vi "Get Tuner Gains.vi"(8 "error in (no error)":errorcluster, 11 "DeviceRefnum":u64) -> (0 "error out":errorcluster, 2 "Supported Gains":dbl[](array[numeric]), 3 "DeviceRefnum Out":u64)   [LabVIEW 2014]
doc: "Get a list of gains supported by the tuner."
panel:
  in  "Gains Buffer":i32[](array[numeric])
  out "function return":i32
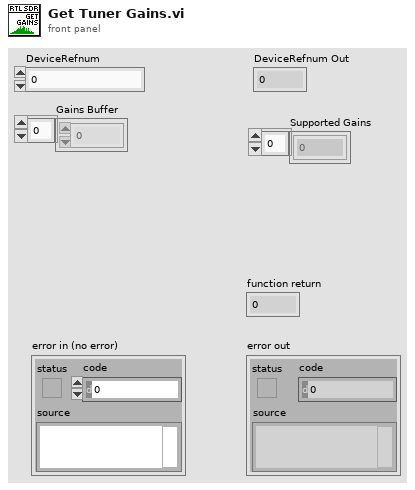
[diagram p1: front panel]
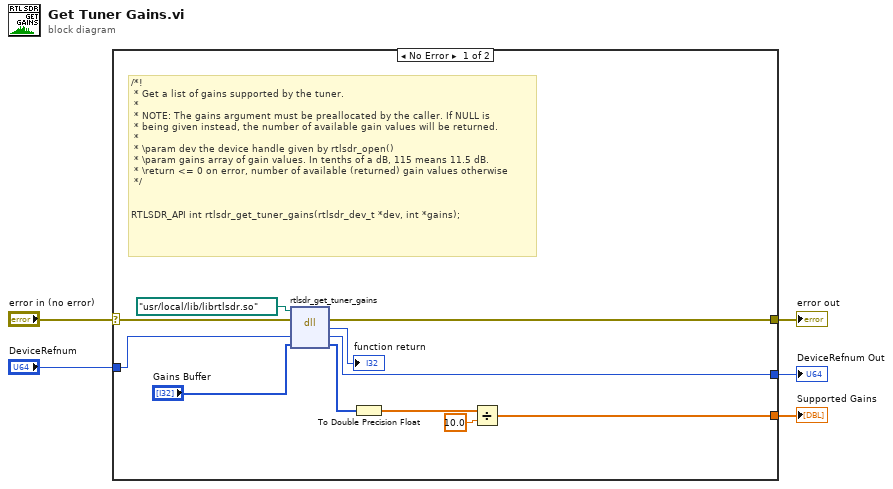
[diagram p0: block diagram]
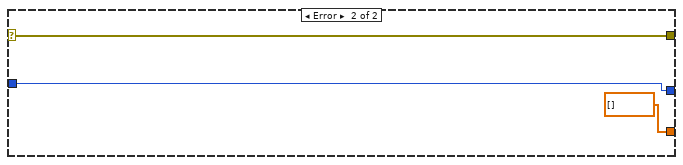
[diagram p2: hidden frame]
diagram:
  n1 = case shown="No Error" "error in (no error)" {
    selector: "error in (no error)" -> [w6 w19]
    tunnel: [w15 w19] -> w5
    tunnel: "DeviceRefnum" -> [w13 w18]
    tunnel: [w11 w18] -> w3
    tunnel: [w7 dbl[] []] -> w2
    frame No Error {
      # "/*!\n * Get a list of gains supported by the tuner.\n *\n * NOTE: The gains argument must be preallocated by the caller. If NULL is\n * being given instead, the number of available gain values will be returned.\n *\n * \\param dev the device handle given by rtlsdr_open()\n * \\param gains array of gain values. In tenths of a dB, 115 means 11.5 dB.\n * \\return <= 0 on error, number of available (returned) gain values otherwise\n */\n\n\nRTLSDR_API int rtlsdr_get_tuner_gains(rtlsdr_dev_t *dev, int *gains);"
      n2 = dll-call lib="C:/Program Files (x86)/National Instruments/LabVIEW 2016/user.lib/rtlsdr/rtlsdr.*" fn="rtlsdr_get_tuner_gains"(path in=path "/usr/local/lib/librtlsdr.so", error in=w6, "DeviceRefnum"=w13, "Gains"="Gains Buffer") -> (error out=w15:errorcluster, "return type"=→"function return":i32, "DeviceRefnum"=w11:u64, "Gains"=w8:i32[])  [unwired: 1 in, 1 out]
      n3 = To Double Precision Float(number=w8) -> (double precision float=w10:dbl[])
      n4 = Divide(x=w10, y=10.0) -> (x/y=w7:dbl[])
    }
    frame Error {
    }
  }
  "error out" <- w5
  "DeviceRefnum Out" <- w3
  "Supported Gains" <- w2
